vi "CSV_Setup_Data_Append.vi"(8 "input cluster":T2={"system"={"info"={"menuSelect"=0, "version"=0, "serial"="Test Sample", "captureActive"=FALSE, "captureBegin"=FALSE, "emptyAndRefill"=FALSE}, "userInfo"={"operatorName"="", "date"=timestamp(2713993200 s since 1904-01-01)}, "camera"={"exposureTime"=0, "aperture"=enum."Item 0", "framerate"=0, "framerateMax"=10, "legacyAttributes"=FALSE}}, "connections"={"arduino"={"connection"="MRJ", "status"=FALSE, "openState"=FALSE, "emptyStart"=0}, "pump"={"connection"="MRJ", "status"=FALSE, "command"="", "dispenseSpeed"=100, "flushSize"=100}, "camera"={"cam1"={"connection"="", "status"=FALSE}, "cam2"={"connection"="", "status"=FALSE}}}, "queue"={"process"={"cam1"=refnum, "cam2"=refnum, "queueSize"=0}, "save"={"cam1"=refnum, "cam2"=refnum, "queueSize"=0}, "overloadThreshold"=0}, "imageProcess"={"cam1"={"preAllocation"={"image"="Station", "originalDisplay"="Station", "originalRgb"="Station", "binary"="Station", "save"="Station", "calibrationFull"=refnum, "calibrationDetect"=refnum}, "calibration"={"pathFull"=path "C:/Users/au540322/Desktop/IHS_Project/images/Debris/Debris_0/Debris_0_2019_06_01-23-32-49-686.PNG", "pathDetect"=path "C:/Users/au540322/Desktop/IHS_Project/images/Debris/Debris_0/Debris_0_2019_06_01-23-32-49-686.PNG", "ROI"={"Left"=0, "Top"=0, "Right"=0, "Bottom"=0, "Rotation"=0.0}}}, "cam2"={"preAllocation"={"image"=refnum, "originalDisplay"=refnum, "originalRgb"=refnum, "binary"=refnum, "save"=refnum, "calibrationFull"=refnum, "calibrationDetect"=refnum}, "calibration"={"pathFull"=path "C:/Users/au540322/Desktop/IHS_Project/images/Debris/Debris_0/Debris_0_2019_06_01-23-32-49-686.PNG", "pathDetect"=path "C:/Users/au540322/Desktop/IHS_Project/images/Debris/Debris_0/Debris_0_2019_06_01-23-32-49-686.PNG", "ROI"={"Left"=0, "Top"=0, "Right"=0, "Bottom"=0, "Rotation"=0.0}}}, "process"={"planeExtract"=refnum, "planeSubtract"=refnum, "cropMask"=refnum}, "detection"={"sampleTimeout"=1, "sizeThreshold"=500, "detectionRegionPct"=0.0}}, "sampleData"={"sampleId"="", "projectId"="", "voucherID"="", "speciesName"="", "collectionDate"=timestamp(2713993200 s since 1904-01-01), "sampleStation"="", "location"="", "lat"=0.0, "lon"=0.0, "determiner"="", "sex"="", "otherNotes"=""}, "Session In"=""} {"sampleData"."collectionDate" format="%<%Y-%m-%d>T"; "imageProcess"."detection"."sizeThreshold" min=1; "imageProcess"."cam2"."calibration"."ROI"."Rotation" format="%.2f"; "imageProcess"."cam2"."calibration"."ROI"."Left" scale=0.0..1024.0; "imageProcess"."cam2"."calibration"."ROI"."Right" scale=0.0..1024.0; "imageProcess"."cam1"."calibration"."ROI"."Rotation" format="%.2f"; "imageProcess"."cam1"."calibration"."ROI"."Left" scale=0.0..1024.0; "imageProcess"."cam1"."calibration"."ROI"."Right" scale=0.0..1024.0; "queue"."overloadThreshold" min=1; "queue"."save"."queueSize" min=1; "queue"."process"."queueSize" min=1; "connections"."pump"."flushSize" min=1; "connections"."pump"."dispenseSpeed" min=1; "system"."camera"."framerateMax" min=1; "system"."userInfo"."date" format="%<%Y-%m-%dT%H:%M:%S+%z>T"; "system"."info"."version" items=["Standard", "XL"]; "system"."info"."menuSelect" items=["Session Data", "Extended Setup", "Buffer", "Camera", "Dispenser", "Stats", "Connections"]}, 9 "summaryData":T1, 10 "Sample Name":string, 11 "Image path":string) -> (3 "Sample Name dup.":string)   [LabVIEW 2022 SP3]
uses:
  controls/Data.ctl
  <vilib>/userdefined/High Color/IMAQdx.ctl
  <vilib>/vision/Image Controls.llb/IMAQ Image.ctl
  <vilib>/Utility/file.llb/Write Delimited Spreadsheet (string).vi
panel:
  out "string":string
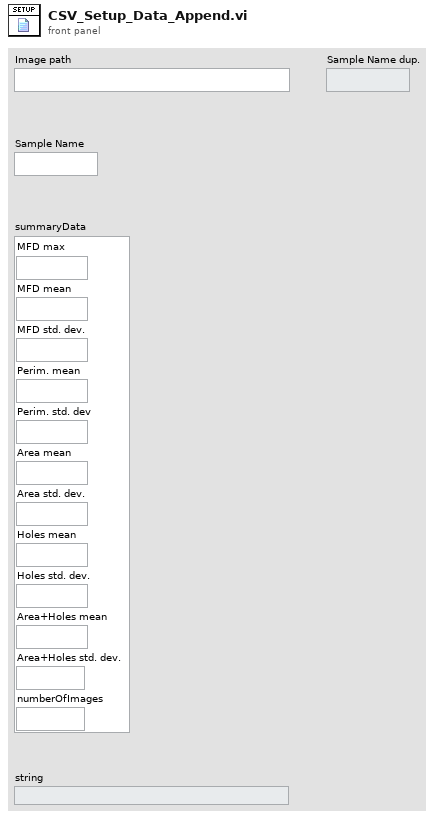
[diagram p1: front panel]
types:
  T1 = cluster{"MFD max":string, "MFD mean":string, "MFD std. dev.":string, "Perim. mean":string, "Perim. std. dev":string, "Area mean":string, "Area std. dev.":string, "Holes mean":string, "Holes std. dev.":string, "Area+Holes mean":string, "Area+Holes std. dev.":string, "numberOfImages":string}
  T2 = typedef "Data.ctl" = cluster{"system":cluster{"info":cluster{"menuSelect":u16, "version":u16, "serial":string, "captureActive":bool, "captureBegin":bool, "emptyAndRefill":bool}, "userInfo":cluster{"operatorName":string, "date":timestamp}, "camera":cluster{"exposureTime":i32, "aperture":enum32{"Item 0", "Item 1", "Item 2", "Item 3"}, "framerate":i32, "framerateMax":i32, "legacyAttributes":bool}}, "connections":cluster{"arduino":cluster{"connection":refnum<visa-resource-name>, "status":bool, "openState":bool, "emptyStart":u32}, "pump":cluster{"connection":refnum<visa-resource-name>, "status":bool, "command":string, "dispenseSpeed":i32, "flushSize":i32}, "camera":cluster{"cam1":cluster{"connection":T3, "status":bool}, "cam2":cluster{"connection":T3, "status":bool}}}, "queue":cluster{"process":cluster{"cam1":refnum<queue>, "cam2":refnum<queue>, "queueSize":i32}, "save":cluster{"cam1":refnum<queue>, "cam2":refnum<queue>, "queueSize":i32}, "overloadThreshold":i32}, "imageProcess":cluster{"cam1":cluster{"preAllocation":cluster{"image":T4, "originalDisplay":T4, "originalRgb":T4, "binary":T4, "save":T4, "calibrationFull":T4, "calibrationDetect":T4}, "calibration":cluster{"pathFull":path, "pathDetect":path, "ROI":T5}}, "cam2":cluster{"preAllocation":cluster{"image":T4, "originalDisplay":T4, "originalRgb":T4, "binary":T4, "save":T4, "calibrationFull":T4, "calibrationDetect":T4}, "calibration":cluster{"pathFull":path, "pathDetect":path, "ROI":T5}}, "process":cluster{"planeExtract":T4, "planeSubtract":T4, "cropMask":T4}, "detection":cluster{"sampleTimeout":i32, "sizeThreshold":i32, "detectionRegionPct":dbl}}, "sampleData":cluster{"sampleId":string, "projectId":string, "voucherID":string, "speciesName":string, "collectionDate":timestamp, "sampleStation":string, "location":string, "lat":dbl, "lon":dbl, "determiner":string, "sex":string, "otherNotes":string}, "Session In":T3}
  T3 = typedef "IMAQdx.ctl" = refnum<k21>
  T4 = typedef "IMAQ Image.ctl" = refnum<image>
  T5 = typedef "IMAQ Rectangle" = cluster{"Left":i32, "Top":i32, "Right":i32, "Bottom":i32, "Rotation":dbl}
  T6 = cluster{"sampleId":string, "projectId":string, "voucherID":string, "speciesName":string, "collectionDate":timestamp, "sampleStation":string, "location":string, "lat":dbl, "lon":dbl, "determiner":string, "sex":string, "otherNotes":string}
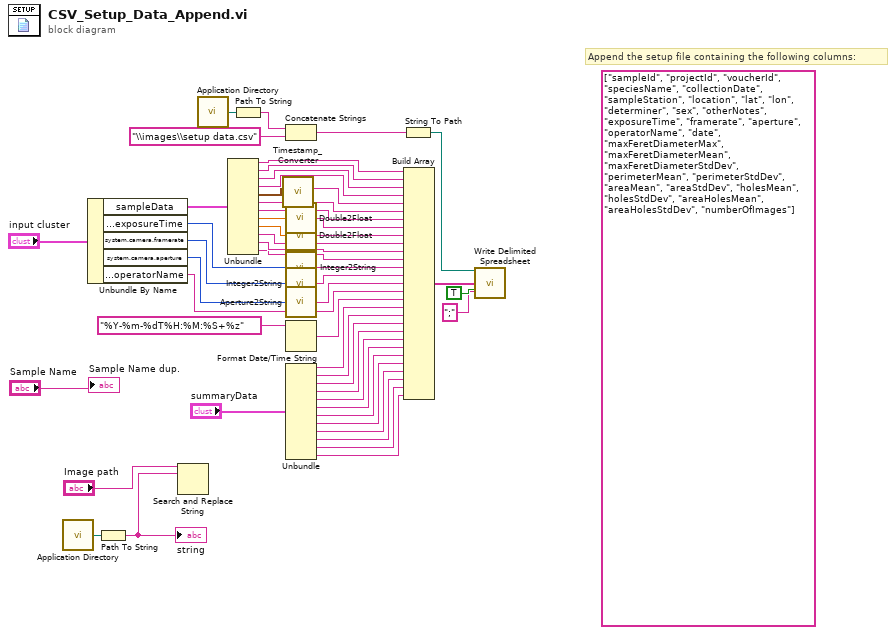
[diagram p0: block diagram]
diagram:
  (unwired) string[] ["sampleId", "projectId", "voucherId", "speciesName", "collectionDate", "sampleStation", "location", "lat", "lon", "determiner", "sex", "otherNotes", "exposureTime", "framerate", "aperture", "operatorName", "date", "maxFeretDiameterMax", "maxFeretDiameterMean", "maxFeretDiameterStdDev", "perimeterMean", "perimeterStdDev", "areaMean", "areaStdDev", "holesMean", "holesStdDev", "areaHolesMean", "areaHolesStdDev", "numberOfImages"]
  # "Append the setup file containing the following columns:"
  n1 = call <vilib>:"Application Directory.vi"() -> ("Application Directory"=w44:path)
  n2 = Unbundle By Name("input cluster") -> ("sampleData"=w38:T6, "system.camera.exposureTime"=w18:i32, "system.camera.framerate"=w22:i32, "system.camera.aperture"=w20:enum32{"Item 0", "Item 1", "Item 2", "Item 3"}, "system.userInfo.operatorName"=w5:string)
  n3 = Path To String(path=w44) -> (string=w42:string)
  "string" <- w42
  n4 = Search and Replace String(input string="Image path", search string=w42) -> ()  [unwired: 6 in, 4 out]
  n5 = call <vilib>:"Application Directory.vi"() -> ("Application Directory"=w48:path)
  n6 = Unbundle(w38) -> ("sampleId"=w37:string, "projectId"=w36:string, "voucherID"=w35:string, "speciesName"=w34:string, "collectionDate"=w33:timestamp, "sampleStation"=w31:string, "location"=w30:string, "lat"=w29:dbl, "lon"=w27:dbl, "determiner"=w25:string, "sex"=w24:string, "otherNotes"=w23:string)
  n7 = Path To String(path=w48) -> (string=w47:string)
  n8 = call "Timestamp_Converter.vi"("Date"=w33) -> ("Date string"=w32:string)  [unwired: 7 in, 1 out]
  n9 = Concatenate Strings(w47, "\\images\\setup data.csv") -> (w45:string)
  n10 = call "Double2Float.vi"("float"=w29) -> ("string"=w28:string)  [unwired: 14 in]
  n11 = call "Double2Float.vi"("float"=w27) -> ("string"=w26:string)  [unwired: 14 in]
  n12 = call "Integer2String.vi"("integer"=w18) -> ("String"=w17:string)  [unwired: 14 in]
  n13 = call "Integer2String.vi"("integer"=w22) -> ("String"=w21:string)  [unwired: 14 in]
  n14 = call "Aperture2String.vi"("aperture"=w20) -> ("String"=w19:string)  [unwired: 14 in]
  n15 = Format Date/Time String(time format string (%c)="%Y-%m-%dT%H:%M:%S+%z") -> (date/time string=w4:string)  [unwired: 2 in]
  n16 = Unbundle("summaryData") -> ("MFD max"=w16:string, "MFD mean"=w15:string, "MFD std. dev."=w14:string, "Perim. mean"=w13:string, "Perim. std. dev"=w12:string, "Area mean"=w11:string, "Area std. dev."=w10:string, "Holes mean"=w9:string, "Holes std. dev."=w8:string, "Area+Holes mean"=w7:string, "Area+Holes std. dev."=w6:string, "numberOfImages"=w2:string)
  n17 = String To Path(string=w45) -> (path=w41:path)
  n18 = Build Array(w37, w36, w35, w34, w32, w31, w30, w28, w26, w25, w24, w23, w17, w21, w19, w5, w4, w16, w15, w14, w13, w12, w11, w10, w9, w8, w7, w6, w2) -> (w39:string[])
  n19 = call-poly <vilib>:"Write Delimited Spreadsheet.vi"("file path (dialog if empty)"=w41, "1D data"=w39, "append to file? (new file:F)"=TRUE, "delimiter (\\t)"=";" ("delimiter (\\t)")) -> ()  [unwired: 10 in, 2 out]
  "Sample Name dup." <- "Sample Name"
